vi "Clear Diagram.vi"(8 "error in (no error)":errorcluster, 11 "top lvl diag in":refnum<vi>) -> (0 "error out":errorcluster, 3 "top lvl diag out":refnum<vi>)   [LabVIEW 2016]
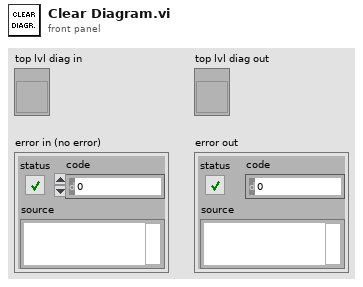
[diagram p1: front panel]
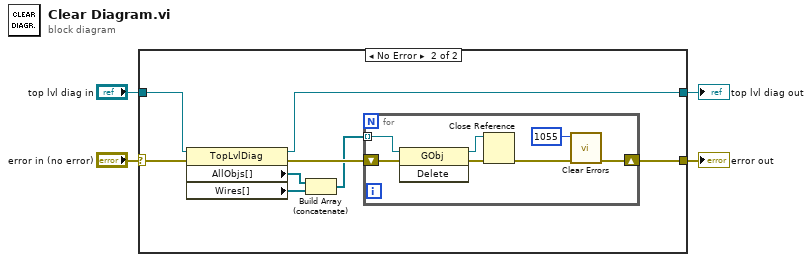
[diagram p0: block diagram]
diagram:
  n1 = case shown="No Error" "error in (no error)" {
    selector: "error in (no error)" -> [w6 w7]
    tunnel: [w5 w10] -> w4
    tunnel: "top lvl diag in" -> [w5 w9]
    tunnel: [w6 w8] -> w1
    frame Error {
    }
    frame No Error {
      n2 = property class="TopLvlDiag"(reference=w9, error in=w7) -> (reference out=w10:refnum<vi>, error out=w14:errorcluster, "AllObjs[]"=w11:refnum<vi>[], "Wires[]"=w12:refnum<vi>[])
      n3 = Build Array (concatenate)(w11, w12) -> (w13:refnum<vi>[])
      n4 = for {
        tunnel: w13 -> [w18] mode=indexing
        shift-right: [w16] -> w8
        shift-left: w14 -> [w21]
        n5 = invoke class="GObj" method="Delete"(reference=w18, error in=w21) -> (reference out=w17:refnum<vi>, error out=w20:errorcluster)  [unwired: 1 in, 1 out]
        n6 = Close Reference(reference=w17, error in (no error)=w20) -> (error out=w19:errorcluster)
        n7 = call <vilib>:"Clear Errors.vi"("error in (no error)"=w19, "specific error code to clear (0: all)"=1055) -> ("error out"=w16:errorcluster)  [unwired: 4 in, 1 out]
      }
    }
  }
  "top lvl diag out" <- w4
  "error out" <- w1
